vi "motionProfileUpdatePath.vi"(10 "Pathname":string="BLANK") -> (2 "Output Path Points":T1[](array[typedef]))   [LabVIEW 2018]
uses:
  <vilib>/Rock Robotics/WPI/ThirdParty/Phoenix-LabVIEW/Motor Controller/Controls/CTRE_Phoenix_MotorControl_MotionProfileTrajectoryPoint.ctl
  driveShifterEnum.ctl
  <vilib>/Utility/file.llb/Read Delimited Spreadsheet (DBL).vi
  <vilib>/Rock Robotics/WPI/ThirdParty/Phoenix-LabVIEW/Motor Controller/Closed Loop/Motion Profile/CTRE_Phoenix_MotorControl_BufferedTrajectoryPointStream_WriteAll.vi
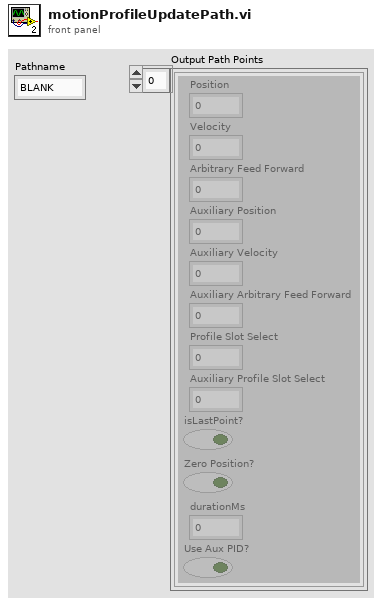
[diagram p1: front panel]
types:
  T1 = typedef "CTRE_Phoenix_MotorControl_MotionProfileTrajectoryPoint.ctl" = cluster{"Position":dbl, "Velocity":dbl, "Arbitrary Feed Forward":dbl, "Auxiliary Position":dbl, "Auxiliary Velocity":dbl, "Auxiliary Arbitrary Feed Forward":dbl, "Profile Slot Select":i32, "Auxiliary Profile Slot Select":i32, "isLastPoint?":bool, "Zero Position?":bool, "durationMs":u32, "Use Aux PID?":bool}
  T2 = typedef "driveShifterEnum.ctl" = enum16{"Low", "High"}
  T3 = enum16{"Inches -> Sensor Units", "Sensor Units -> Inches"}
  T4 = typedef "CTRE_Phoenix_MotorControl_BufferedTrajectoryPointStream_DeviceRef.ctl" = cluster{"Handle":u64, "Library Path":path}
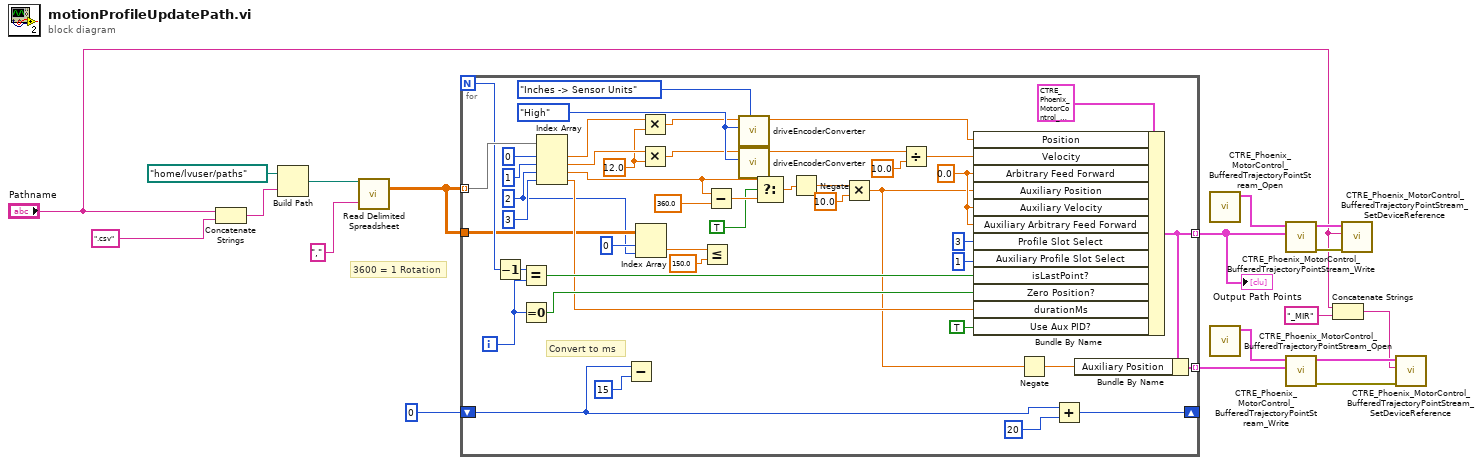
[diagram p0: block diagram]
diagram:
  # "3600 = 1 Rotation"
  n1 = Concatenate Strings("Pathname", ".csv") -> (w14:string)
  n2 = Build Path(base path=path "/home/lvuser/paths", name or relative path=w14) -> (appended path=w9:path)
  n3 = call-poly <vilib>:"Read Delimited Spreadsheet.vi"("file path (dialog if empty)"=w9, "delimiter (\\t)"="," ("delimiter (\\t)")) -> ("all rows"=w1:dbl[][])  [unwired: 8 in, 5 out]
  n4 = for {
    N -> [w58]
    tunnel: w1 -> [w63] mode=indexing
    tunnel: [w32] -> w11 mode=indexing
    shift-right: [w46] -> _
    shift-left: u32 0 ("durationMs") -> [w44]
    tunnel: [w31] -> w2 mode=indexing
    tunnel: w1 -> [w28]
    i -> [w53]
    w38 = driveShifterEnum."High" ("Gear Setting")
    w33 = 12.0 ("y")
    w37 = T3."Inches -> Sensor Units" ("Conversion Direction")
    w26 = 2 ("index")
    w62 = 0.0 ("Arbitrary Feed Forward")
    # "Convert to ms"
    n5 = Decrement(x=w58) -> (x-1=w52:i32)
    n6 = Equal?(x=w52, y=w53) -> (x = y?=w59:bool)
    n7 = Equal To 0?(x=w53) -> (x = 0?=w57:bool)
    n8 = Index Array(array=w63, index #1=0 ("index"), index #2=1 ("index"), index #3=w26, index #4=3 ("index")) -> (element #1=w42:dbl, element #2=w39:dbl, element #3=w22:dbl, element #4=w36:dbl)
    n9 = Subtract(x=w44, y=u32 15) -> ()  [unwired: 1 out]
    n10 = Index Array(array=w28, index (row)=0, index (col)=w26) -> (element=w24:dbl)
    n11 = Multiply(x=w42, y=w33) -> (x*y=w35:dbl)
    n12 = Multiply(x=w39, y=w33) -> (x*y=w34:dbl)
    n13 = Less Or Equal?(x=w24, y=150.0) -> ()  [unwired: 1 out]
    n14 = Subtract(x=w22, y=360.0) -> (x-y=w21:dbl)
    n15 = call "driveEncoderConverter.vi"("Conversion Direction"=w37, "Gear Setting"=w38, "Input"=w35) -> ("Output"=w41:dbl)  [unwired: 8 in]
    n16 = call "driveEncoderConverter.vi"("Conversion Direction"=w37, "Gear Setting"=w38, "Input"=w34) -> ("Output"=w40:dbl)  [unwired: 8 in]
    n17 = Select(t=w22, s=TRUE, f=w21) -> (s? t:f=w25:dbl)
    n18 = Negate(x=w25) -> (-x=w47:dbl)
    n19 = Multiply(x=w47, y=10.0) -> (x*y=w29:dbl)
    n20 = Divide(x=w40, y=10.0) -> (x/y=w54:dbl)
    n21 = Bundle By Name(cluster=T1 {"Position"=0.0, "Velocity"=0.0, "Arbitrary Feed Forward"=0.0, "Auxiliary Position"=0.0, "Auxiliary Velocity"=0.0, "Auxiliary Arbitrary Feed Forward"=0.0, "Profile Slot Select"=0, "Auxiliary Profile Slot Select"=0, "isLastPoint?"=FALSE, "Zero Position?"=FALSE, "durationMs"=0, "Use Aux PID?"=FALSE} ("Trajectory Point"), "Position"=w41, "Velocity"=w54, "Arbitrary Feed Forward"=w62, "Auxiliary Position"=w29, "Auxiliary Velocity"=w62, "Auxiliary Arbitrary Feed Forward"=w62, "Profile Slot Select"=3, "Auxiliary Profile Slot Select"=1, "isLastPoint?"=w59, "Zero Position?"=w57, "durationMs"=w36, "Use Aux PID?"=TRUE) -> (w32:T1)
    n22 = Negate(x=w29) -> (-x=w30:dbl)
    n23 = Add(x=w44, y=u32 20) -> (x+y=w46:u32)
    n24 = Bundle By Name(cluster=w32, "Auxiliary Position"=w30) -> (w31:T1)
  }
  "Output Path Points" <- w11
  n25 = call <vilib>:"CTRE_Phoenix_MotorControl_BufferedTrajectoryPointStream_Open.vi"() -> ("BufferedTrajectoryPointStream_DevRef"=w16:T4)  [unwired: 10 in, 1 out]
  n26 = call <vilib>:"CTRE_Phoenix_MotorControl_BufferedTrajectoryPointStream_Open.vi"() -> ("BufferedTrajectoryPointStream_DevRef"=w8:T4)  [unwired: 10 in, 1 out]
  n27 = call-poly <vilib>:"CTRE_Phoenix_MotorControl_BufferedTrajectoryPointStream_Write.vi"("Motion Profile Trajectory Point Array"=w11, "BufferedTrajectoryPointStream_DevRef"=w16) -> ("error out"=w18:errorcluster, "BufferedTrajectoryPointStream_DevRef"=w17:T4)  [unwired: 8 in]
  n28 = call-poly <vilib>:"CTRE_Phoenix_MotorControl_BufferedTrajectoryPointStream_Write.vi"("Motion Profile Trajectory Point Array"=w2, "BufferedTrajectoryPointStream_DevRef"=w8) -> ("error out"=w6:errorcluster, "BufferedTrajectoryPointStream_DevRef"=w7:T4)  [unwired: 8 in]
  n29 = Concatenate Strings("Pathname", "_MIR" ("string")) -> (w3:string)
  n30 = call <vilib>:"CTRE_Phoenix_MotorControl_BufferedTrajectoryPointStream_SetDeviceReference.vi"("error in (no error)"=w18, "refnum name"="Pathname", "BufferedTrajectoryPointStream_DevRef"=w17) -> ()  [unwired: 7 in, 2 out]
  n31 = call <vilib>:"CTRE_Phoenix_MotorControl_BufferedTrajectoryPointStream_SetDeviceReference.vi"("error in (no error)"=w6, "refnum name"=w3, "BufferedTrajectoryPointStream_DevRef"=w7) -> ()  [unwired: 7 in, 2 out]
